vi "Write Channels.vi"(8 "error in (no error)":errorcluster, 10 "Channels":string[](array[string]), 11 "CryoCoolerAVC in":refnum<class "CryoCoolerAVC.lvclass">) -> (0 "error out":errorcluster, 3 "CryoCoolerAVC out":refnum<class "CryoCoolerAVC.lvclass">)   [LabVIEW 2022 SP3, in "CryoCoolerAVC.lvclass"]
uses:
  CryoCoolerAVC.lvclass
  CryoCoolerAVC.lvclass/CryoCoolerAVC.ctl
  Cryo Cooler.lvclass
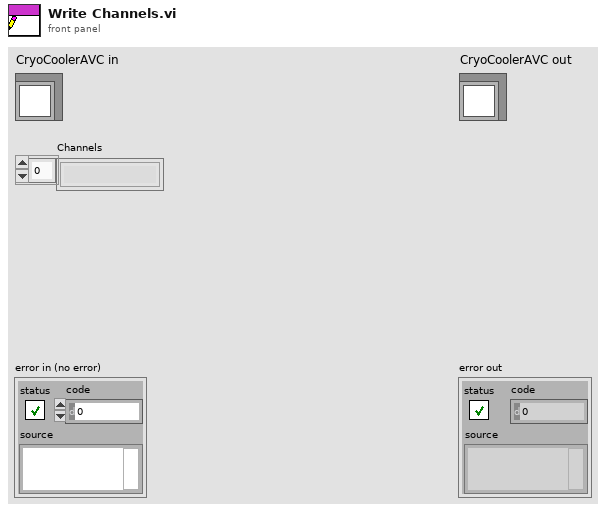
[diagram p1: front panel]
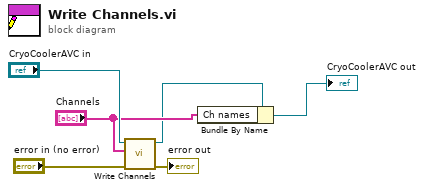
[diagram p0: block diagram]
diagram:
  n1 = call-parent "Write Channels.vi"("error in (no error)"="error in (no error)", "Channels"="Channels", "Cryo Cooler in"="CryoCoolerAVC in") -> ("error out"=→"error out":errorcluster, "Cryo Cooler out"=w2:refnum<class "CryoCoolerAVC.lvclass">)  [unwired: 7 in]
  n2 = Bundle By Name(cluster=w2, "Ch names"="Channels") -> (→"CryoCoolerAVC out":refnum<class "CryoCoolerAVC.lvclass">)
